vi "Manual Override.vi"(8 "Override":enum32{"None", "Intake", "Eject", "STOP"}(ring), 10 "Position GO":bool, 11 "Auto CMD":T1) -> (2 "Position GO Out":bool, 3 "OverRide Command Out":T1)   [LabVIEW 2020, in "Grabber_ACT.lvlib"]
uses:
  Grabber_ACT.lvlib
  Cluster_CMD_ACT_Data.ctl
  Shared Code/TypeDefs/ENUM_Grabber_CMD_Mode Select.ctl
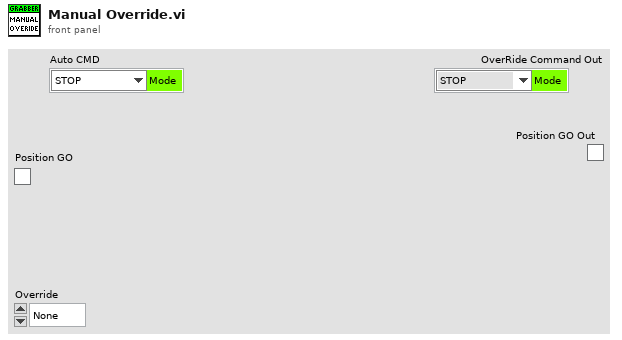
[diagram p1: front panel]
types:
  T1 = typedef "Grabber_ACT.lvlib/Cluster_CMD_ACT_Data.ctl" = cluster{"Mode":T2}
  T2 = typedef "ENUM_Grabber_CMD_Mode Select.ctl" = enum16{"STOP", "Intake", "Eject"}
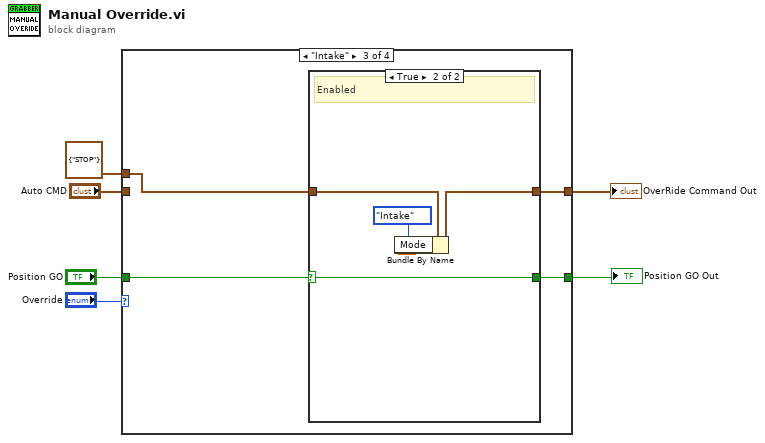
[diagram p0: block diagram]
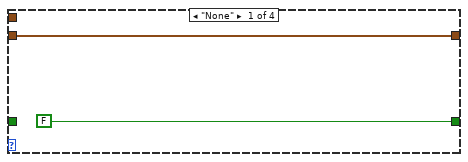
[diagram p2: hidden frame]
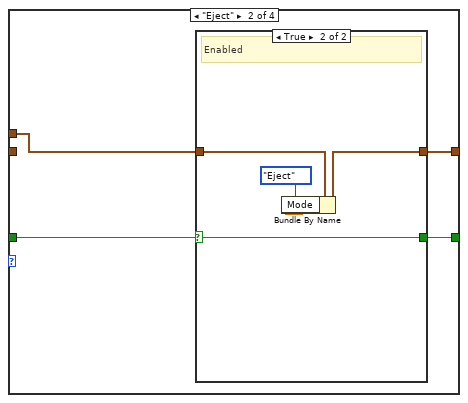
[diagram p3: hidden frame]
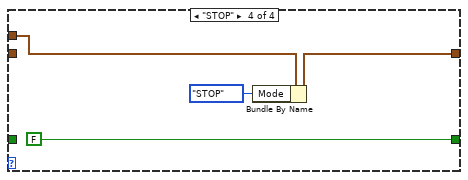
[diagram p6: hidden frame]
diagram:
  n1 = case shown="\"Intake\"" "Override" {
    tunnel: [w7 w11 w21 w30] -> w6
    tunnel: T1 {"Mode"=enum."STOP"} ("CMD_ExtendTemplate_Data 3") -> [_ w12 w22 w29]
    tunnel: "Position GO" -> [_ w10 w20 _]
    tunnel: [FALSE w9 w19 FALSE] -> w4
    tunnel: "Auto CMD" -> [w7 _ _ _]
    frame "None" {
    }
    frame "Eject" {
      (unwired) 0.0 ("Velocity")
      n2 = case shown="True" w10 {
        selector: w10 -> [w13 w16]
        tunnel: w12 -> [w14 w18]
        tunnel: [w14 w17] -> w11
        tunnel: [w13 w16] -> w9
        frame False {
          # "Disabled"
        }
        frame True {
          # "Enabled"
          n3 = Bundle By Name(cluster=w18, "Mode"=ENUM_Grabber_CMD_Mode_Select."Eject") -> (w17:T1)
        }
      }
    }
    frame "Intake" {
      (unwired) 0.0 ("Velocity")
      n4 = case shown="True" w20 {
        selector: w20 -> [w23 w26]
        tunnel: w22 -> [w24 w28]
        tunnel: [w24 w27] -> w21
        tunnel: [w23 w26] -> w19
        frame False {
          # "Disabled"
        }
        frame True {
          # "Enabled"
          n5 = Bundle By Name(cluster=w28, "Mode"=ENUM_Grabber_CMD_Mode_Select."Intake") -> (w27:T1)
        }
      }
    }
    frame "STOP" {
      n6 = Bundle By Name(cluster=w29, "Mode"=ENUM_Grabber_CMD_Mode_Select."STOP") -> (w30:T1)
    }
  }
  "OverRide Command Out" <- w6
  "Position GO Out" <- w4
